vi "Read_statuscode_ini.vi"(8 "Error In":errorcluster, 11 "Input status selection":i32) -> (0 "Error Out":errorcluster, 2 "StatusCode path":path, 3 "Status_selected":string)   [LabVIEW 2017]
doc: "This subVI fetches all the error description from the ErrorCodes.ini file\n \n\\\\..\\UltraSonic_Test_Scripts\\Generic_Common\\Webserver\\ErrorCodes.ini\n\nNote: User can modify the error descriptions in ErrorCodes.ini file, located in above path"
uses:
  <vilib>/Utility/config.llb/Read Key (String).vi
  <vilib>/Utility/config.llb/NI_LVConfig.lvlib
panel:
  out "Error discription":string[](array[string])
  out "Keys in ini":string[](array[string])
  # "READ FROM STATUS CODE INI FILE"
  # "ERROR"
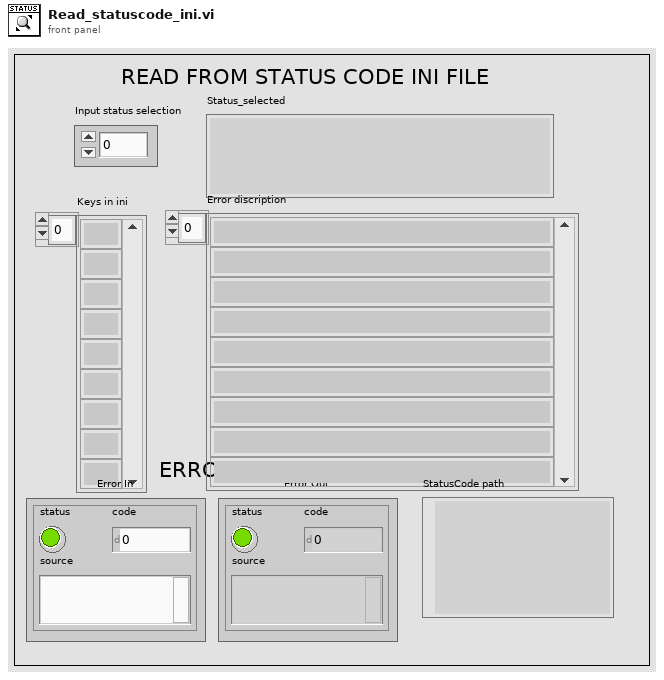
[diagram p1: front panel]
types:
  T1 = typedef "NI_LVConfig.lvlib/Config Data RefNum.ctl" = refnum<k1>
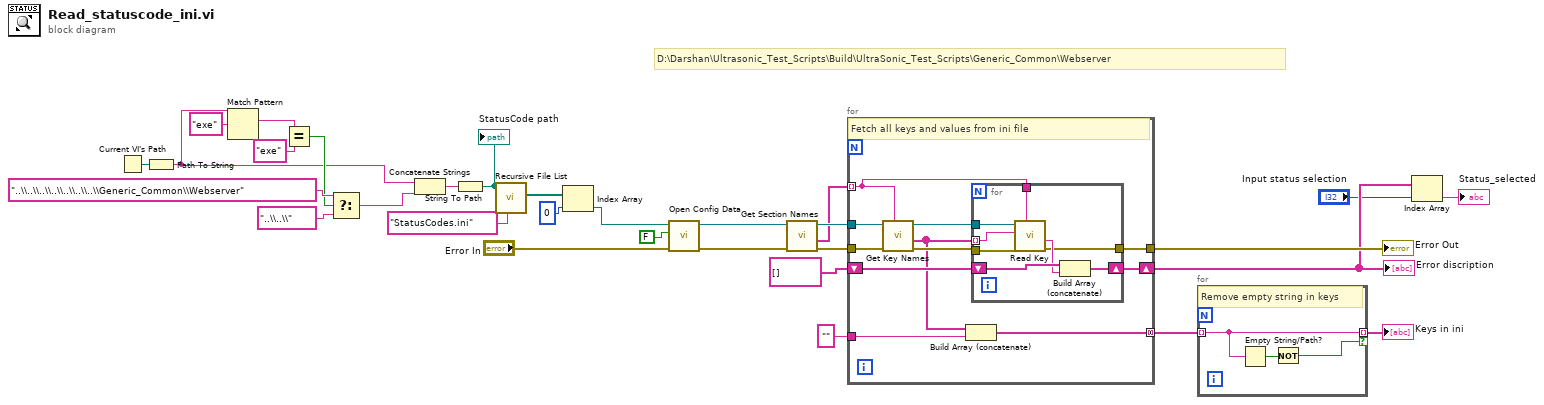
[diagram p0: block diagram]
diagram:
  # "D:\\Darshan\\Ultrasonic_Test_Scripts\\Build\\UltraSonic_Test_Scripts\\Generic_Common\\Webserver"
  n1 = Current VI's Path() -> (path=w4:path)
  n2 = Path To String(path=w4) -> (string=w3:string)
  n3 = Match Pattern(string=w3, regular expression="exe") -> (match substring=w8:string)  [unwired: 1 in, 3 out]
  n4 = Equal?(x=w8, y="exe") -> (x = y?=w6:bool)
  n5 = Select(t="..\\..\\..\\..\\..\\..\\..\\Generic_Common\\Webserver" ("string"), s=w6, f="..\\..\\" ("string")) -> (s? t:f=w2:string)
  n6 = Concatenate Strings(w3, w2) -> (w1:string)
  n7 = String To Path(string=w1) -> (path=w18:path)
  "StatusCode path" <- w18
  n8 = call <vilib>:"Recursive File List.vi"("pattern"="StatusCodes.ini", "Folder Path"=w18) -> ("All Files in Dir"=w16:path[])  [unwired: 5 in, 4 out]
  n9 = Index Array(array=w16, index=0) -> (element=w14:path)
  n10 = call <vilib>:"Open Config Data.vi"("error in (no error)"="Error In", "create file if necessary (T)"=FALSE ("create file if necessary? (T)"), "configuration file path"=w14) -> ("error out"=w27:errorcluster, "refnum"=w29:T1)  [unwired: 6 in, 1 out]
  n11 = call <vilib>:"Get Section Names.vi"("error in (no error)"=w27, "refnum"=w29) -> ("error out"=w26:errorcluster, "section names"=w25:string[], "refnum out"=w28:T1)  [unwired: 7 in]
  n12 = for {
    tunnel: w28 -> [w39]
    tunnel: w26 -> [w38]
    tunnel: w25 -> [w37] mode=indexing
    shift-right: [w36] -> w13
    shift-left: string[] [] -> [w35]
    tunnel: "" -> [w33]
    tunnel: [w32] -> w22 mode=concatenating
    tunnel: [w31] -> w19
    # "Fetch all keys and values from ini file"
    n13 = call <vilib>:"Get Key Names.vi"("section"=w37, "error in (no error)"=w38, "refnum"=w39) -> ("error out"=w40:errorcluster, "key names"=w34:string[], "refnum out"=w41:T1)  [unwired: 5 in, 1 out]
    n14 = Build Array (concatenate)(w34, w33) -> (w32:string[])
    n15 = for {
      tunnel: w34 -> [w45] mode=indexing
      tunnel: w41 -> [w49]
      tunnel: w40 -> [w48]
      shift-right: [w47] -> w36
      shift-left: w35 -> [w44]
      tunnel: w37 -> [w46]
      tunnel: [w42] -> w31
      n16 = call-poly <vilib>:"Read Key.vi"("section"=w46, "error in (no error)"=w48, "key"=w45, "refnum"=w49) -> ("error out"=w42:errorcluster, "value"=w43:string)  [unwired: 2 in, 4 out]
      n17 = Build Array (concatenate)(w44, w43) -> (w47:string[])
    }
  }
  "Error Out" <- w19
  "Error discription" <- w13
  n18 = for {
    tunnel: w22 -> [w51] mode=indexing
    tunnel: [w51] -> w21 mode=indexing if=w50
    # "Remove empty string in keys"
    n19 = Empty String/Path?(string/path=w51) -> (empty?=w52:bool)
    n20 = Not(x=w52) -> (.not. x?=w50:bool)
  }
  "Keys in ini" <- w21
  n21 = Index Array(array=w13, index="Input status selection") -> (element=→"Status_selected":string)
